vi "TCP-Get Error Message.vi"(11 "error in (no error)":errorcluster) -> (4 "Message":string, 15 "error out":errorcluster)   [LabVIEW 2020]
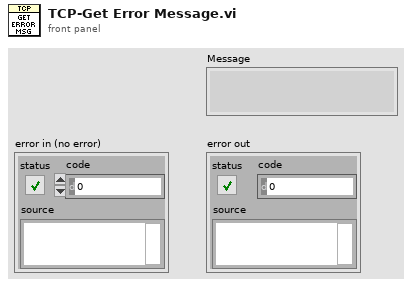
[diagram p1: front panel]
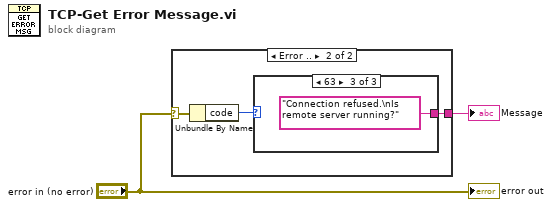
[diagram p0: block diagram]
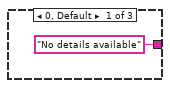
[diagram p3: hidden frame]
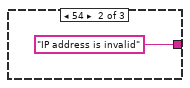
[diagram p4: hidden frame]
diagram:
  n1 = case shown="Error .." "error in (no error)" {
    selector: "error in (no error)" -> [_ w5]
    tunnel: [_ w3] -> w1
    frame No Error {
    }
    frame Error {
      n2 = Unbundle By Name(w5) -> ("code"=w4:i32)
      n3 = case shown="63" w4 {
        tunnel: ["No details available" "IP address is invalid" "Connection refused.\nIs remote server running?"] -> w3
        frame 0, Default {
        }
        frame 54 {
        }
        frame 63 {
        }
      }
    }
  }
  "Message" <- w1
  "error out" <- "error in (no error)"
